vi "Configure Manual Mode.vi"(0 "VISA resource name":refnum<visa-resource-name>, 1 "Voltage Low Limit (0 V)":dbl min=0.0 max=400.0 format="%.1f", 2 "Voltage High Limit (300 V)":dbl=300.0 min=0.0 max=400.0 format="%.1f", 5 "Enable Over Current Fold Back (F:Disable)":bool, 7 "Start Angle (0)":i32 min=0 max=359, 9 "End Angle: (0)":i32 min=0 max=359, 11 "error in (no error)":errorcluster, 12 "Frequency Low Limit (40 Hz)":dbl=40.0 min=0.0 max=500.0 format="%.1f", 13 "Frequency High Limit (500 Hz)":dbl=500.0 min=0.0 max=500.0 format="%.1f") -> (4 "VISA resource name out":refnum<visa-resource-name>, 15 "error out":errorcluster)   [LabVIEW 2020, in "eec 6700.lvlib"]
doc: "Sets the instrument to manual mode and configures required parameters in the power source instrument.\n\nIn manual mode, the instrument can be configured with a particular power sourcesettings and testing parameters"
uses:
  <instrlib>/EEC6700LV-driver/eec 6700.lvlib
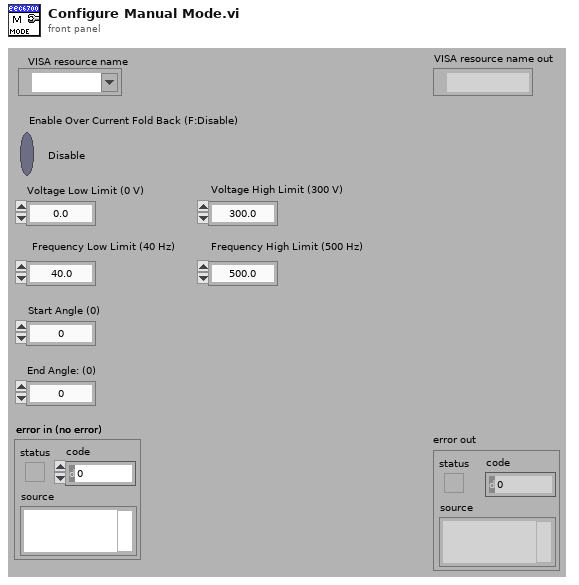
[diagram p1: front panel]
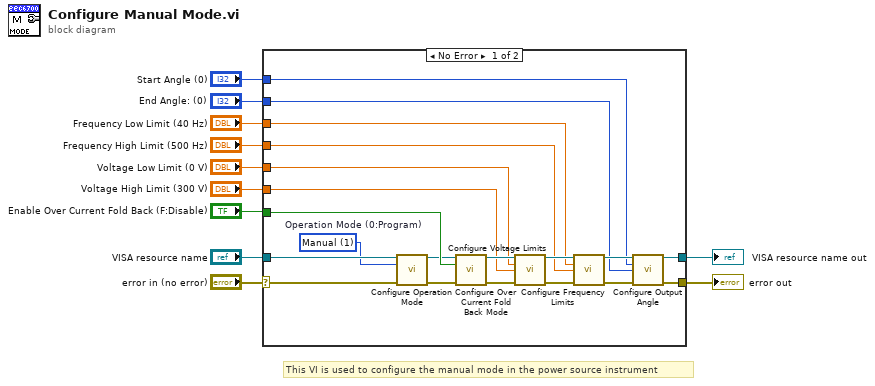
[diagram p0: block diagram]
diagram:
  # "This VI is used to configure the manual mode in the power source instrument"
  n1 = case shown="No Error" "error in (no error)" {
    selector: "error in (no error)" -> [w31 w32]
    tunnel: "VISA resource name" -> [w30 w33]
    tunnel: [w19 w33] -> w9
    tunnel: [w20 w32] -> w8
    tunnel: "Enable Over Current Fold Back (F:Disable)" -> [w29 _]
    tunnel: "Voltage Low Limit (0 V)" -> [w18 _]
    tunnel: "Voltage High Limit (300 V)" -> [w17 _]
    tunnel: "Frequency Low Limit (40 Hz)" -> [w16 _]
    tunnel: "Frequency High Limit (500 Hz)" -> [w15 _]
    tunnel: "Start Angle (0)" -> [w14 _]
    tunnel: "End Angle: (0)" -> [w13 _]
    frame No Error {
      w12 = u16 1 items=["Program", "Manual"]  # Operation Mode (0:Program)
      n2 = call <instrlib>:"Configure Operation Mode.vi"("VISA resource name"=w30, "Operation Mode (0:Program)"=w12, "error in (no error)"=w31) -> ("VISA resource name out"=w28:refnum<visa-resource-name>, "error out"=w27:errorcluster)  [unwired: 11 in]
      n3 = call <instrlib>:"Configure Over Current Fold Back Mode.vi"("VISA resource name"=w28, "Enable Over Current Fold Back (F:Disable)"=w29, "error in (no error)"=w27) -> ("VISA resource name out"=w22:refnum<visa-resource-name>, "error out"=w21:errorcluster)  [unwired: 11 in]
      n4 = call <instrlib>:"Configure Voltage Limits.vi"("VISA resource name"=w22, "Voltage Low Limit (0 V)"=w18, "Voltage High Limit (300 V)"=w17, "error in (no error)"=w21) -> ("VISA resource name out"=w26:refnum<visa-resource-name>, "error out"=w25:errorcluster)  [unwired: 10 in]
      n5 = call <instrlib>:"Configure Frequency Limits.vi"("VISA resource name"=w26, "Frequency Low Limit (40 Hz)"=w16, "Frequency High Limit (500 Hz)"=w15, "error in (no error)"=w25) -> ("VISA resource name out"=w24:refnum<visa-resource-name>, "error out"=w23:errorcluster)  [unwired: 10 in]
      n6 = call <instrlib>:"Configure Output Angle.vi"("VISA resource name"=w24, "Start Angle (0)"=w14, "End Angle: (0)"=w13, "error in (no error)"=w23) -> ("VISA resource name out"=w19:refnum<visa-resource-name>, "error out"=w20:errorcluster)  [unwired: 10 in]
    }
    frame Error {
    }
  }
  "error out" <- w8
  "VISA resource name out" <- w9
